vi "CAN.vi"() -> ()   [LabVIEW 2020]
uses:
  Global_Variable/Global.vi
  Global_Variable/A180648.vi
  Libraries/ZLG_CAN/ZLG_CAN.lvlib
panel:
  in  "CAN 通道":u32(ring) items=["0", "1"]
  in  "索引":u32(ring) items=["0", "1", "2", "3", "4", "5", "6", "7", "8"]
  in  "设备类型":u32(ring)=27 items=["PCI5121"=1, "PCI9810"=2, "USBCAN1"=3, "USBCAN2"=4, "PCI9820"=5, "PCI5110"=7, "PC104CAN"=11, "CANETUDP"=12, "PCI9840B"=14, "PC104C2"=15, "PCI9820I"=16, "CANETTCP"=17, "PCIE9221"=24, "PCI5010U"=19, "USBCAN_E_U"=20, "USBCAN_2E_U"=21, "PCI5020U"=22, "PCIE9120I"=27, "PCIE9110I"=28, "PCIE9140I"=29]
  in  "Stop":bool
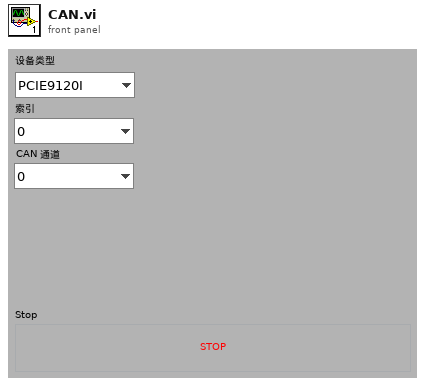
[diagram p1: front panel]
types:
  T1 = cluster{"波特率":u32, "ID":u32, "帧类型":enum8{"标准帧", "扩展帧"}, "帧格式":enum16{"数据帧", "远程帧"}, "周期(ms)":u32}
  T2 = typedef "ZLG_CAN.lvlib/Start_CAN (Reply Payload)--cluster.ctl" = cluster{"Success":bool, "Start_CAN_error":errorcluster}
  T3 = cluster{u8, u8, "y":u8, "y":u8, "y":u8, "y":u8, "y":u8, "y":u8}
  T4 = cluster{"y":u8, "y":u8, "y":u8, u8, u8, "y":u8, "y":u8, "y":u8}
  T5 = cluster{"[0]":u8, "[1]":u8, "[2]":u8, "[3]":u8, "[4]":u8, "[5]":u8, "[6]":u8, "[7]":u8}
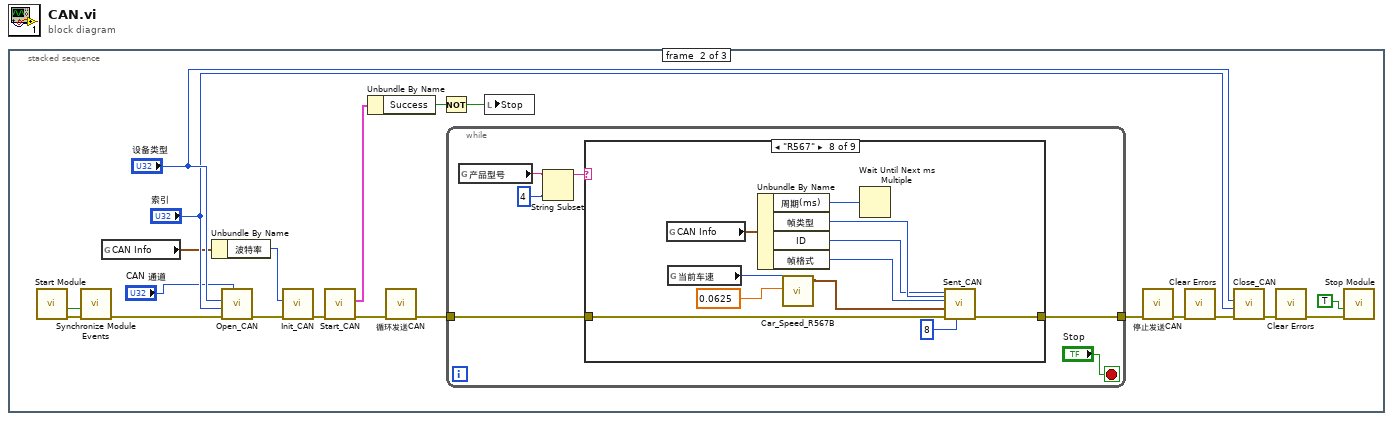
[diagram p0: block diagram]
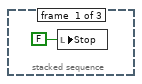
[diagram p2: hidden frame]
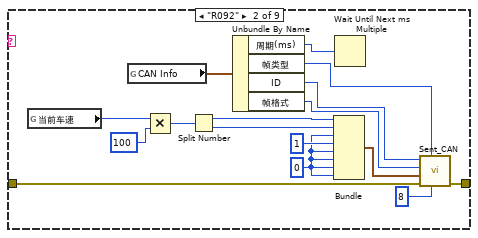
[diagram p4: hidden frame]
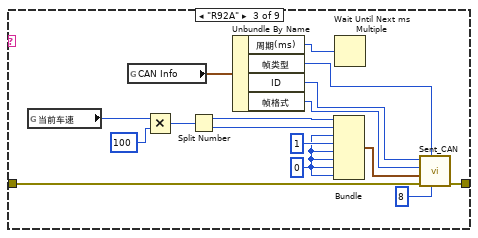
[diagram p5: hidden frame]
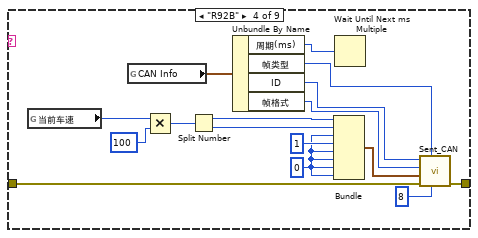
[diagram p6: hidden frame]
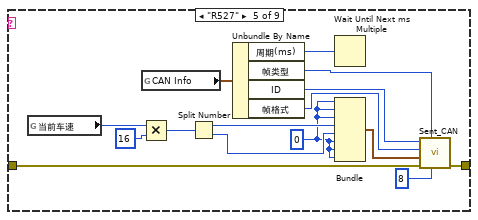
[diagram p7: hidden frame]
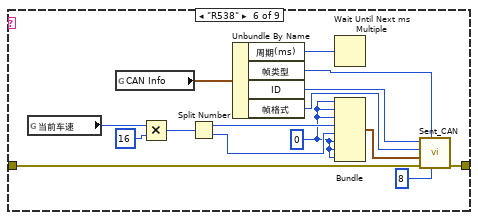
[diagram p8: hidden frame]
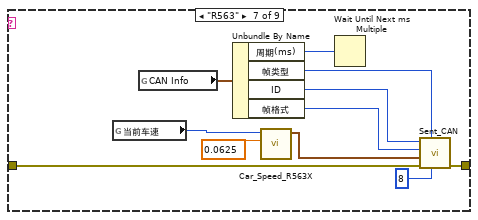
[diagram p9: hidden frame]
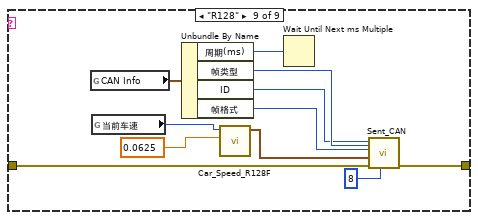
[diagram p10: hidden frame]
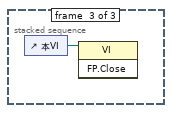
[diagram p11: hidden frame]
diagram:
  n1 = stacked-sequence {
    frame #0 {
      n2 = local write "Stop"(FALSE ("Stop")) -> ()
    }
    frame #1 {
      n3 = call "Start Module.vi"() -> ("error out"=w22:errorcluster, "Wait for Event Sync?"=w21:bool)  [unwired: 8 in, 2 out]
      n4 = call "Synchronize Module Events.vi"("error in (no error)"=w22, "Wait for Event Sync?"=w21) -> ("error out"=w20:errorcluster)  [unwired: 9 in]
      n5 = global read "Global.vi" "CAN Info"() -> (w7:T1)
      n6 = Unbundle By Name(w7) -> ("波特率"=w12:u32)
      n7 = call "Open_CAN.vi"("CAN 通道"="CAN 通道", "error in (no error)"=w20, "索引"="索引", "设备类型"="设备类型") -> ("error out"=w17:errorcluster)  [unwired: 7 in]
      n8 = call "Init_CAN.vi"("error in (no error)"=w17, "波特率"=w12) -> ("error out"=w13:errorcluster)  [unwired: 9 in]
      n9 = call "Start_CAN.vi"("error in (no error)"=w13) -> ("error out"=w6:errorcluster, "Reply Payload"=w15:T2)  [unwired: 8 in, 1 out]
      n10 = Unbundle By Name(w15) -> ("Success"=w14:bool)
      n11 = call "循环发送CAN.vi"("错误输入"=w6) -> ("错误输出"=w5:errorcluster)  [unwired: 10 in]
      n12 = Not(x=w14) -> (.not. x?=w2:bool)
      n13 = while {
        tunnel: w5 -> [w28]
        tunnel: [w27] -> w4
        stop <- "Stop" stop-if-true
        n14 = global read "Global.vi" "产品型号"() -> (w25:string)
        n15 = String Subset(string=w25, length (rest)=4 ("长度（剩余）")) -> (substring=w23:string)  [unwired: 1 in]
        n16 = case shown="\"R567\"" w23 {
          tunnel: w28 -> [w29 w45 w61 w77 w92 w107 w118 w129 w140]
          tunnel: [w29 w44 w60 w76 w91 w106 w117 w128 w139] -> w27
          frame "假", Default {
          }
          frame "R092" {
            w30 = u8 0 ("y")
            n17 = global read "A180648.vi" "当前车速"() -> (w31:u16)
            n18 = global read "Global.vi" "CAN Info"() -> (w32:T1)
            n19 = Multiply(x=w31, y=u16 100) -> (x*y=w42:u16)
            n20 = Split Number(x=w42) -> (hi(x)=w41:u8, lo(x)=w40:u8)
            n21 = Unbundle By Name(w32) -> ("周期(ms)"=w36:u32, "帧类型"=w34:enum8{"标准帧", "扩展帧"}, "ID"=w33:u32, "帧格式"=w35:enum16{"数据帧", "远程帧"})
            n22 = Bundle(w41, w40, "y"=w30, "y"=u8 1, "y"=w30, "y"=w30, "y"=w30, "y"=w30) -> (w38:T3)  [unwired: 1 in]
            n23 = Wait Until Next ms Multiple(millisecond multiple=w36) -> ()  [unwired: 1 out]
            n24 = call "Sent_CAN.vi"("帧长度"=u8 8, "帧类型"=w34, "error in (no error)"=w45, "帧数据"=w38, "帧格式"=w35, "ID"=w33) -> ("error out"=w44:errorcluster)  [unwired: 5 in]
          }
          frame "R92A" {
            w46 = u8 0 ("y")
            n25 = global read "A180648.vi" "当前车速"() -> (w47:u16)
            n26 = global read "Global.vi" "CAN Info"() -> (w48:T1)
            n27 = Multiply(x=w47, y=u16 100) -> (x*y=w58:u16)
            n28 = Split Number(x=w58) -> (hi(x)=w57:u8, lo(x)=w56:u8)
            n29 = Unbundle By Name(w48) -> ("周期(ms)"=w52:u32, "帧类型"=w50:enum8{"标准帧", "扩展帧"}, "ID"=w49:u32, "帧格式"=w51:enum16{"数据帧", "远程帧"})
            n30 = Bundle(w57, w56, "y"=w46, "y"=u8 1, "y"=w46, "y"=w46, "y"=w46, "y"=w46) -> (w54:T3)  [unwired: 1 in]
            n31 = Wait Until Next ms Multiple(millisecond multiple=w52) -> ()  [unwired: 1 out]
            n32 = call "Sent_CAN.vi"("帧长度"=u8 8, "帧类型"=w50, "error in (no error)"=w61, "帧数据"=w54, "帧格式"=w51, "ID"=w49) -> ("error out"=w60:errorcluster)  [unwired: 5 in]
          }
          frame "R92B" {
            w62 = u8 0 ("y")
            n33 = global read "A180648.vi" "当前车速"() -> (w63:u16)
            n34 = global read "Global.vi" "CAN Info"() -> (w64:T1)
            n35 = Multiply(x=w63, y=u16 100) -> (x*y=w74:u16)
            n36 = Split Number(x=w74) -> (hi(x)=w73:u8, lo(x)=w72:u8)
            n37 = Unbundle By Name(w64) -> ("周期(ms)"=w68:u32, "帧类型"=w66:enum8{"标准帧", "扩展帧"}, "ID"=w65:u32, "帧格式"=w67:enum16{"数据帧", "远程帧"})
            n38 = Bundle(w73, w72, "y"=w62, "y"=u8 1, "y"=w62, "y"=w62, "y"=w62, "y"=w62) -> (w70:T3)  [unwired: 1 in]
            n39 = Wait Until Next ms Multiple(millisecond multiple=w68) -> ()  [unwired: 1 out]
            n40 = call "Sent_CAN.vi"("帧长度"=u8 8, "帧类型"=w66, "error in (no error)"=w77, "帧数据"=w70, "帧格式"=w67, "ID"=w65) -> ("error out"=w76:errorcluster)  [unwired: 5 in]
          }
          frame "R527" {
            w78 = u8 0 ("y")
            n41 = global read "A180648.vi" "当前车速"() -> (w81:u16)
            n42 = Multiply(x=w81, y=u16 16) -> (x*y=w89:u16)
            n43 = global read "Global.vi" "CAN Info"() -> (w82:T1)
            n44 = Split Number(x=w89) -> (hi(x)=w80:u8, lo(x)=w79:u8)
            n45 = Unbundle By Name(w82) -> ("周期(ms)"=w86:u32, "帧类型"=w84:enum8{"标准帧", "扩展帧"}, "ID"=w83:u32, "帧格式"=w85:enum16{"数据帧", "远程帧"})
            n46 = Wait Until Next ms Multiple(millisecond multiple=w86) -> ()  [unwired: 1 out]
            n47 = Bundle("y"=w78, "y"=w78, "y"=w78, w80, w79, "y"=w78, "y"=w78, "y"=w78) -> (w88:T4)  [unwired: 1 in]
            n48 = call "Sent_CAN.vi"("帧长度"=u8 8, "帧类型"=w84, "error in (no error)"=w92, "帧数据"=w88, "帧格式"=w85, "ID"=w83) -> ("error out"=w91:errorcluster)  [unwired: 5 in]
          }
          frame "R538" {
            w93 = u8 0 ("y")
            n49 = global read "A180648.vi" "当前车速"() -> (w96:u16)
            n50 = global read "Global.vi" "CAN Info"() -> (w97:T1)
            n51 = Multiply(x=w96, y=u16 16) -> (x*y=w104:u16)
            n52 = Split Number(x=w104) -> (hi(x)=w95:u8, lo(x)=w94:u8)
            n53 = Unbundle By Name(w97) -> ("周期(ms)"=w101:u32, "帧类型"=w99:enum8{"标准帧", "扩展帧"}, "ID"=w98:u32, "帧格式"=w100:enum16{"数据帧", "远程帧"})
            n54 = Wait Until Next ms Multiple(millisecond multiple=w101) -> ()  [unwired: 1 out]
            n55 = Bundle("y"=w93, "y"=w93, "y"=w93, w95, w94, "y"=w93, "y"=w93, "y"=w93) -> (w103:T4)  [unwired: 1 in]
            n56 = call "Sent_CAN.vi"("帧长度"=u8 8, "帧类型"=w99, "error in (no error)"=w107, "帧数据"=w103, "帧格式"=w100, "ID"=w98) -> ("error out"=w106:errorcluster)  [unwired: 5 in]
          }
          frame "R563" {
            n57 = global read "A180648.vi" "当前车速"() -> (w109:u16)
            n58 = global read "Global.vi" "CAN Info"() -> (w111:T1)
            n59 = Unbundle By Name(w111) -> ("周期(ms)"=w115:u32, "帧类型"=w113:enum8{"标准帧", "扩展帧"}, "ID"=w112:u32, "帧格式"=w114:enum16{"数据帧", "远程帧"})
            n60 = call "Car_Speed_R563X.vi"("精度"=0.0625, "车速"=w109) -> ("报文"=w108:T5)  [unwired: 9 in]
            n61 = Wait Until Next ms Multiple(millisecond multiple=w115) -> ()  [unwired: 1 out]
            n62 = call "Sent_CAN.vi"("帧长度"=u8 8, "帧类型"=w113, "error in (no error)"=w118, "帧数据"=w108, "帧格式"=w114, "ID"=w112) -> ("error out"=w117:errorcluster)  [unwired: 5 in]
          }
          frame "R567" {
            n63 = global read "Global.vi" "CAN Info"() -> (w122:T1)
            n64 = global read "A180648.vi" "当前车速"() -> (w121:u16)
            n65 = Unbundle By Name(w122) -> ("周期(ms)"=w126:u32, "帧类型"=w124:enum8{"标准帧", "扩展帧"}, "ID"=w123:u32, "帧格式"=w125:enum16{"数据帧", "远程帧"})
            n66 = call "Car_Speed_R567B.vi"("精度"=0.0625, "车速"=w121) -> ("报文"=w119:T5)  [unwired: 9 in]
            n67 = Wait Until Next ms Multiple(millisecond multiple=w126) -> ()  [unwired: 1 out]
            n68 = call "Sent_CAN.vi"("帧长度"=u8 8, "帧类型"=w124, "error in (no error)"=w129, "帧数据"=w119, "帧格式"=w125, "ID"=w123) -> ("error out"=w128:errorcluster)  [unwired: 5 in]
          }
          frame "R128" {
            n69 = global read "Global.vi" "CAN Info"() -> (w133:T1)
            n70 = global read "A180648.vi" "当前车速"() -> (w131:u16)
            n71 = Unbundle By Name(w133) -> ("周期(ms)"=w137:u32, "帧类型"=w135:enum8{"标准帧", "扩展帧"}, "ID"=w134:u32, "帧格式"=w136:enum16{"数据帧", "远程帧"})
            n72 = call "Car_Speed_R128F.vi"("精度"=0.0625, "车速"=w131) -> ("报文"=w132:T5)  [unwired: 9 in]
            n73 = Wait Until Next ms Multiple(millisecond multiple=w137) -> ()  [unwired: 1 out]
            n74 = call "Sent_CAN.vi"("帧长度"=u8 8, "帧类型"=w135, "error in (no error)"=w140, "帧数据"=w132, "帧格式"=w136, "ID"=w134) -> ("error out"=w139:errorcluster)  [unwired: 5 in]
          }
        }
      }
      n75 = local write "Stop"(w2) -> ()
      n76 = call "停止发送CAN.vi"("错误输入"=w4) -> ("错误输出"=w3:errorcluster)  [unwired: 10 in]
      n77 = call <vilib>:"Clear Errors.vi"("error in (no error)"=w3) -> ("error out"=w8:errorcluster)  [unwired: 5 in, 1 out]
      n78 = call "Close_CAN.vi"("error in (no error)"=w8, "索引"="索引", "设备类型"="设备类型") -> ("error out"=w11:errorcluster)  [unwired: 8 in]
      n79 = call <vilib>:"Clear Errors.vi"("error in (no error)"=w11) -> ("error out"=w9:errorcluster)  [unwired: 5 in, 1 out]
      n80 = call "Stop Module.vi"("error in (no error)"=w9, "Wait for Module to Stop? (F)"=TRUE) -> ()  [unwired: 9 in, 1 out]
    }
    frame #2 {
      n81 = control-ref of="本VI"() -> (w141:refnum<vi>)
      n82 = invoke class="VI" method="FP.Close"(reference=w141) -> ()  [unwired: 2 in, 3 out]
    }
  }
